vi "Load temperature reader Modules.vi"(8 "Error In":errorcluster) -> (0 "Error Out":errorcluster, 2 "Menu control":T1, 3 "Modules":refnum<class "Template Module.lvclass">[](array[class]))   [LabVIEW 2020]
uses:
  LabActor/Template Module/Template Module.lvclass
  LabActor/Controllers/Application Controller/Menu Control.ctl
  LabActor/Instrument Actor/Instrument Actor.lvclass
  opt/github/LabActor/Template Module/Template Module.lvclass
  Temperature reader/temperature reader.lvclass
  opt/github/NHMFL_Core/Libraries/Instruments/Instrument Driver/Instrument Driver.lvclass
  LabActor/Instrument Actor/Instrument Actor.lvclass/Instrument Actor.ctl
  LabActor/Template Module/Template Module.lvclass/Template Module.ctl
  LabActor/Template Module/Write Name.vi
  LabActor/Instrument Actor/Write Instrument driver.vi
  ZI Lockin/ZI Lockin.lvclass
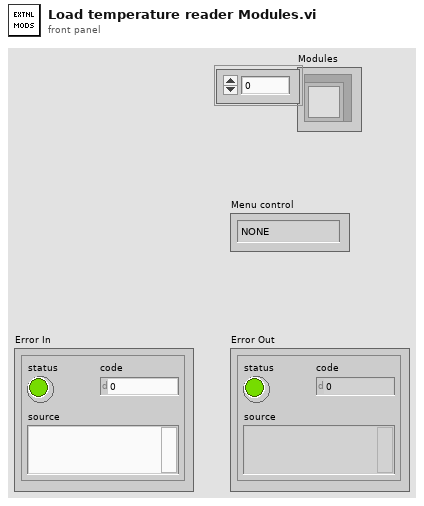
[diagram p1: front panel]
types:
  T1 = typedef "Menu Control.ctl" = enum16{"NONE", "Monitor", "Post-process", "Pulse"}
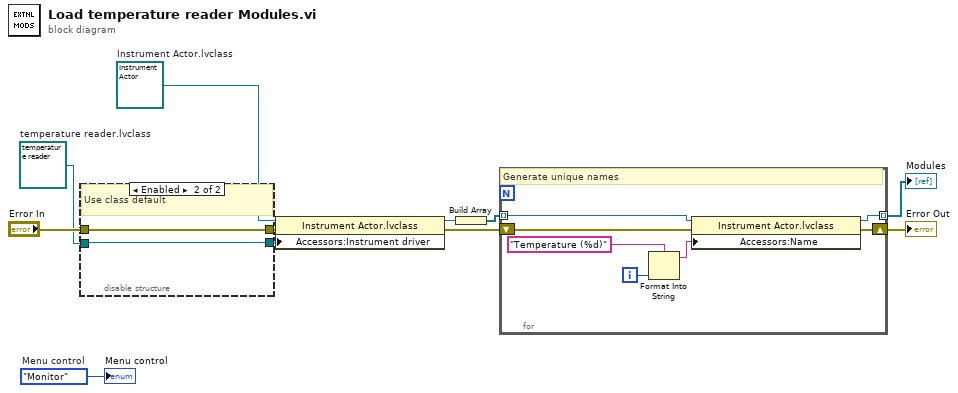
[diagram p0: block diagram]
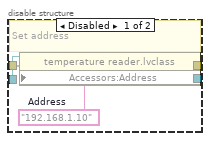
[diagram p2: hidden frame]
diagram:
  w8 = Menu_Control."Monitor"  # Menu control
  w6 = refnum<class "temperature reader.lvclass"> refnum  # temperature reader.lvclass
  w11 = refnum<class "Instrument Actor.lvclass"> refnum  # Instrument Actor.lvclass
  n1 = disable-structure shown="Enabled" {
    disable-tunnel: "Error In" -> [w16 w18]
    disable-tunnel: [w15 w18] -> w7
    disable-tunnel: w6 -> [w14 w17]
    disable-tunnel: [w13 w17] -> w5
    frame Disabled {
      w12 = "192.168.1.10"  # Address
      # "Set address"
      n2 = property class="temperature reader.lvclass"(reference=w14, error in=w16, "Accessors:Address"=w12) -> (reference out=w13:refnum<class "temperature reader.lvclass">, error out=w15:errorcluster)
    }
    frame Enabled {
      # "Use class default"
    }
  }
  n3 = property class="Instrument Actor.lvclass"(reference=w11, error in=w7, "Accessors:Instrument driver"=w5) -> (reference out=w9:refnum<class "Instrument Actor.lvclass">, error out=w3:errorcluster)
  n4 = Build Array(w9) -> (w4:refnum<class "Instrument Actor.lvclass">[])
  n5 = for {
    tunnel: w4 -> [w25] mode=indexing
    shift-right: [w23] -> w1
    shift-left: w3 -> [w24]
    tunnel: [w22] -> w2 mode=indexing
    i -> [w21]
    # "Generate unique names"
    n6 = Format Into String(format string="Temperature (%d)" ("Name"), w21) -> (resulting string=w19:string)  [unwired: 2 in, 1 out]
    n7 = property class="Instrument Actor.lvclass"(reference=w25, error in=w24, "Accessors:Name"=w19) -> (reference out=w22:refnum<class "Instrument Actor.lvclass">, error out=w23:errorcluster)
  }
  "Modules" <- w2
  "Error Out" <- w1
  "Menu control" <- w8
